vi "dialogue--exit_app.vi"(8 "error in (no error)":errorcluster) -> (0 "error out":errorcluster, 3 "T = exit was pressed":bool)   [LabVIEW 2020, in "main.lvlib"]
doc: "Blank VI with error handling."
uses:
  main.lvlib
  PTRL/GUI_tools/Dialogues/Dialogues.lvlib
panel:
  # "Development\ncontrols/indicators useful for development and testing, but which are not outputs of the VI"
  # "Input\nInputs to the VI"
  # "Output\nOutputs of the VI"
  # "Description\n\nBlank VI with error handling case. \n\nSummarize the use of this VI in this space."
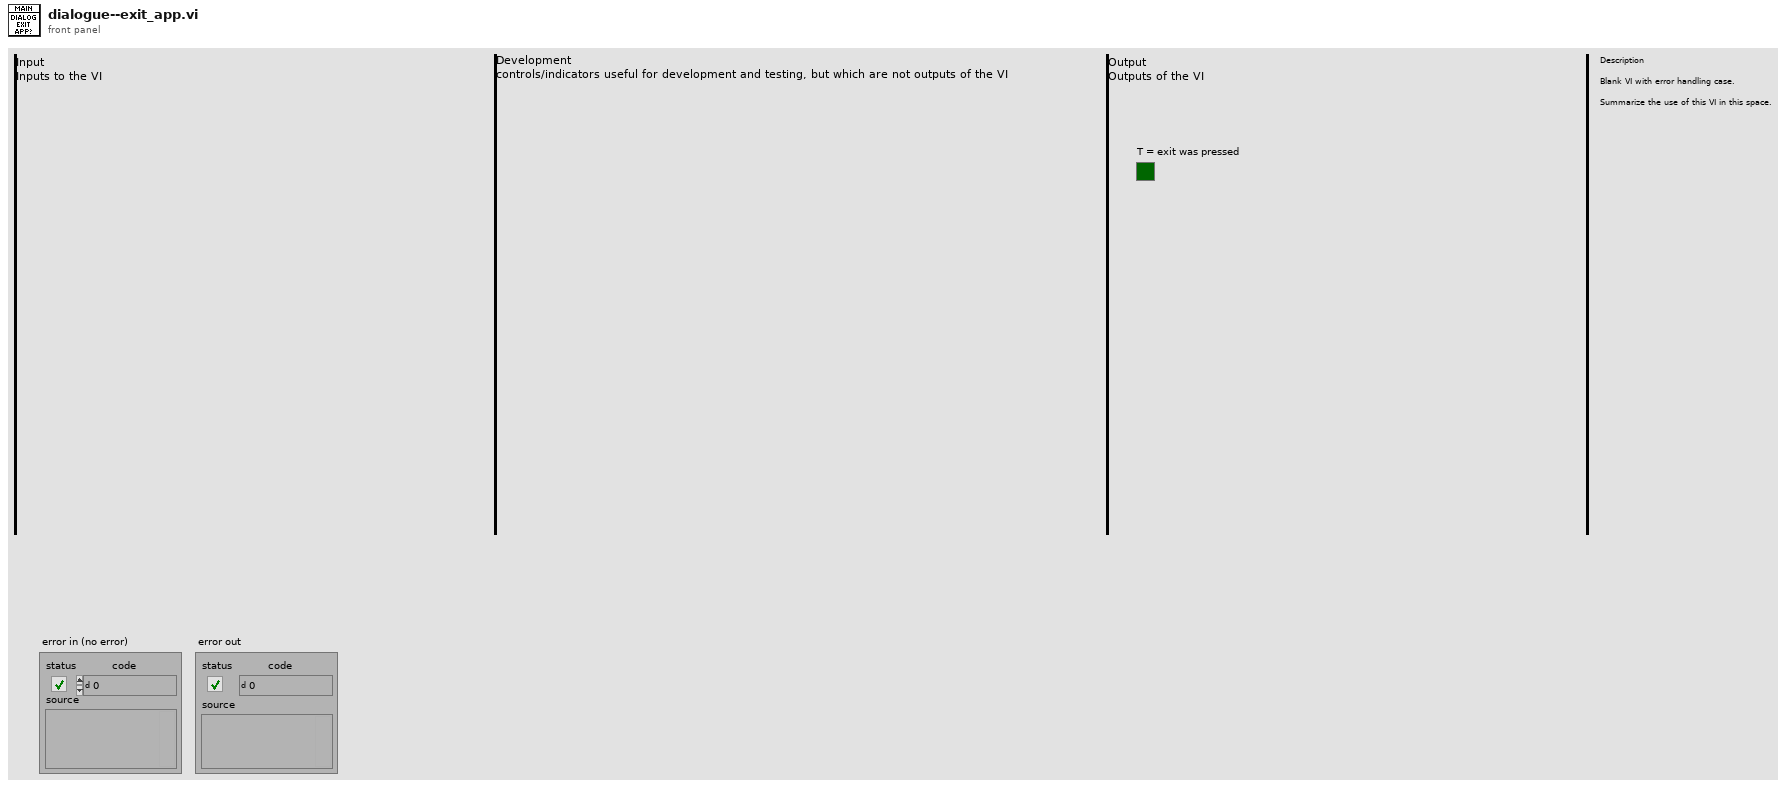
[diagram p1: front panel]
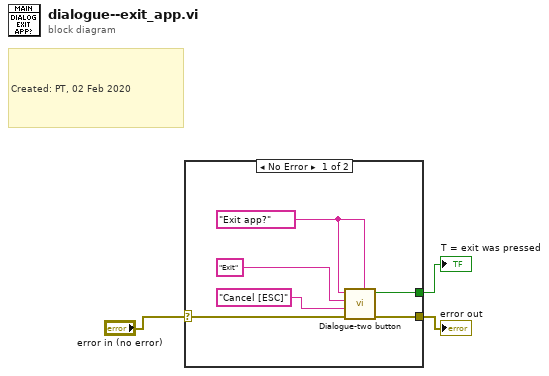
[diagram p0: block diagram]
diagram:
  # "Created: PT, 02 Feb 2020"
  n1 = case shown="No Error" "error in (no error)" {
    selector: "error in (no error)" -> [w9 w10]
    tunnel: [w8 w10] -> w2
    tunnel: [w4 _] -> w1
    frame No Error {
      w7 = "Exit app?" ("VI Title (dflt=\"Dialogue\")")
      n2 = call "Dialogue-two button.vi"("VI Title (dflt=\"Dialogue\")"=w7, "error in (no error)"=w9, "F button name (\"Cancel (ESC)\")"="Cancel [ESC]" ("F button name (\"Cancel (ESC)\")"), "T button name (\"OK\")"="Exit" ("T button name (\"OK\")"), "User Message"=w7) -> ("error out"=w8:errorcluster, "T button?"=w4:bool)  [unwired: 5 in]
    }
    frame Error {
    }
  }
  "error out" <- w2
  "T = exit was pressed" <- w1
